vi "A-H 2500 Cap.vi"(2 "Point #":i32, 3 "Instrument Address":refnum<visa-resource-name>) -> (0 "Stop":bool, 1 "Measurement":dbl[](array[numeric]) format="%.9f")   [LabVIEW 2024]
doc: "Reads Andeen Haegerling Automatic Capacitance bridge and returns the capacitance in pF. Does not use SRQ lines.\nScott Hannahs, F. Bitter National Magnet Lab, May 1993"
panel:
  in  "Return Dissapation":u8(slide) max=5 step=1 scale=0.0..5.0
  in  "AVE TIME":u32(slide)=5 max=15 step=1 scale=0.0..15.0
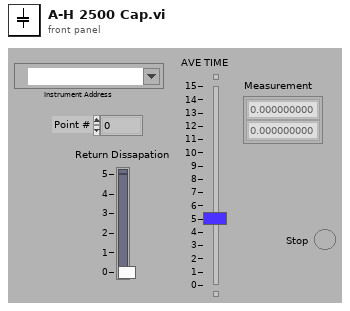
[diagram p1: front panel]
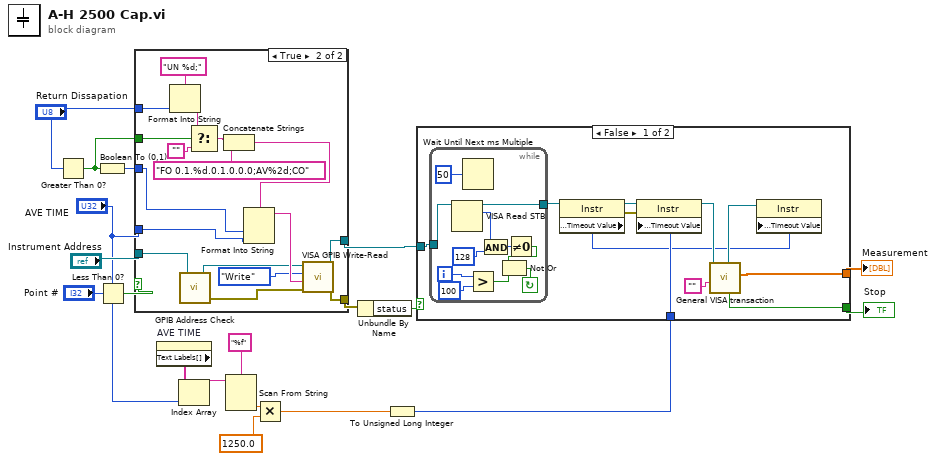
[diagram p0: block diagram]
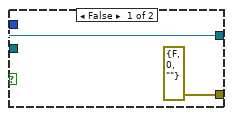
[diagram p2: hidden frame]
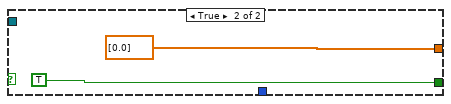
[diagram p3: hidden frame]
diagram:
  n1 = Greater Than 0?(x="Return Dissapation") -> (x > 0?=w10:bool)
  n2 = Boolean To (0,1)(Boolean=w10) -> (0, 1=w9:i16)
  n3 = Less Than 0?(x="Point #") -> (x < 0?=w16:bool)
  n4 = case shown="True" w16 {
    tunnel: [w21 w32] -> w15
    tunnel: "Instrument Address" -> [w21 w34]
    tunnel: [errorcluster {"status"=FALSE, "code"=0, "source"=""} ("error out") w38] -> w18
    tunnel: "AVE TIME" -> [_ w23]
    tunnel: "Return Dissapation" -> [_ w26]
    tunnel: w10 -> [_ w24]
    tunnel: w9 -> [_ w22]
    frame False {
    }
    frame True {
      n5 = Format Into String(format string="UN %d;" ("Input String"), w26) -> (resulting string=w28:string)  [unwired: 2 in, 1 out]
      n6 = call "GPIB Address Check.vi"("Instrument Address"=w34) -> ("dup VISA session"=w33:refnum<visa-resource-name>, "error out"=w37:errorcluster)  [unwired: 1 in, 1 out]
      n7 = Select(t=w28, s=w24, f="") -> (s? t:f=w30:string)
      n8 = Concatenate Strings(w30, "FO 0.1.%d.0.1.0.0.0;AV%2d;CO") -> (w25:string)
      n9 = Format Into String(format string=w25, w22, w23) -> (resulting string=w36:string)  [unwired: 2 in, 1 out]
      n10 = call "VISA GPIB Write-Read.vi"("error in (no error)"=w37, "Command"=w36, "Action"=enum16{"Write", "Read", "Write & Read"}."Write", "VISA resource name"=w33) -> ("error out"=w38:errorcluster, "dup VISA Session"=w32:refnum<visa-resource-name>)  [unwired: 4 in, 2 out]
    }
  }
  n11 = property on="AVE TIME" class="Slide (strict)"() -> ("Text Labels[]"=w3:string[])  [unwired: 2 in, 2 out]
  n12 = Index Array(array=w3, index="AVE TIME") -> (element=w4:string)
  n13 = Scan From String(format string="%f" ("Format String"), input string=w4) -> (output 1=w6:dbl)  [unwired: 3 in, 3 out]
  n14 = Multiply(x=w6, y=1250.0) -> (x*y=w8:dbl)
  n15 = Unbundle By Name(w18) -> ("status"=w19:bool)
  n16 = To Unsigned Long Integer(number=w8) -> (unsigned 32bit integer=w1:u32)
  n17 = case shown="False" w19 {
    tunnel: w15 -> [w46 _]
    tunnel: [w49 dbl[] [0.0]] -> w13
    tunnel: [w48 TRUE ("Stop")] -> w12
    tunnel: w1 -> [w41 _]
    frame False {
      n18 = while {
        tunnel: [w51] -> w43
        tunnel: w46 -> [w50]
        i -> [w58]
        stop <- w56 continue-if-true
        n19 = VISA Read STB(11:w50) -> (2:w52:u16, 3:w51:refnum<visa-resource-name>)  [unwired: 1 in, 1 out]
        n20 = Wait Until Next ms Multiple(millisecond multiple=u32 50) -> ()  [unwired: 1 out]
        n21 = Greater?(x=w58, y=100) -> (0:w55:bool)
        n22 = And(x=w52, y=u16 128) -> (x .and. y?=w53:u16)
        n23 = Not Equal To 0?(x=w53) -> (x != 0?=w54:bool)
        n24 = Not Or(1:w55, 2:w54) -> (0:w56:bool)
      }
      n25 = property class="Instr"(reference=w43) -> (reference out=w44:refnum<visa-resource-name>, error out=w45:errorcluster, "General Settings:Timeout Value"=w39:u32)  [unwired: 1 in]
      n26 = property class="Instr"(reference=w44, error in=w45, "General Settings:Timeout Value"=w41) -> (reference out=w42:refnum<visa-resource-name>)  [unwired: 1 out]
      n27 = call "General VISA transaction.vi"("Command String"="", "VISA Session"=w42) -> ("Measurement"=w49:dbl[], "dup VISA Session"=w40:refnum<visa-resource-name>, "Stop"=w48:bool)  [unwired: 4 in, 3 out]
      n28 = property class="Instr"(reference=w40, "General Settings:Timeout Value"=w39) -> ()  [unwired: 1 in, 2 out]
    }
    frame True {
    }
  }
  "Measurement" <- w13
  "Stop" <- w12
